vi "Variablen Generator.vi"(10 "Numerisch":i32) -> (2 "Verknüpfter String":string)   [LabVIEW 2020, in "FT-IR.lvlib" / "Algebraic Modul.lvlib"]
uses:
  Algebraic Modul.lvlib
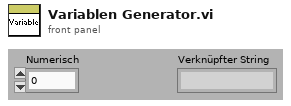
[diagram p1: front panel]
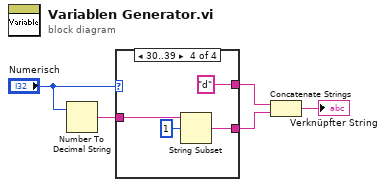
[diagram p0: block diagram]
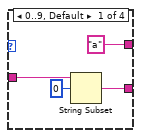
[diagram p2: hidden frame]
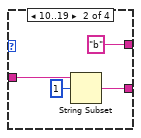
[diagram p3: hidden frame]
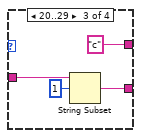
[diagram p4: hidden frame]
diagram:
  n1 = Number To Decimal String(number="Numerisch") -> (decimal integer string=w2:string)  [unwired: 1 in]
  n2 = case shown="30..39" "Numerisch" {
    tunnel: ["a" "b" "c" "d"] -> w5
    tunnel: [w7 w11 w15 w19] -> w4
    tunnel: w2 -> [w6 w10 w14 w18]
    frame 0..9, Default {
      n3 = String Subset(string=w6, offset (0)=0 ("Offset (0)")) -> (substring=w7:string)  [unwired: 1 in]
    }
    frame 10..19 {
      n4 = String Subset(string=w10, offset (0)=1 ("Offset (0)")) -> (substring=w11:string)  [unwired: 1 in]
    }
    frame 20..29 {
      n5 = String Subset(string=w14, offset (0)=1 ("Offset (0)")) -> (substring=w15:string)  [unwired: 1 in]
    }
    frame 30..39 {
      n6 = String Subset(string=w18, offset (0)=1 ("Offset (0)")) -> (substring=w19:string)  [unwired: 1 in]
    }
  }
  n7 = Concatenate Strings(w5, w4) -> (→"Verknüpfter String":string)
